vi "_Test_CRC_Calc.vi"() -> ()   [LabVIEW 2023, in "LP_CRC.lvlib"]
uses:
  LP_CRC.lvlib
panel:
  in  "Frame ID":i32=385
  out "CRC":u8=125 format="%x"
  in  "Data_In":u8[](array[numeric])=[125, 14, 64, 52, 12, 67, 49, 12, 53, 182, 13, 34, 66, 38, 86, 4, 38, 197, 29, 38, 104, 26, 34, 172, 51, 120, 150, 1, 0, 0, 0, 0, 0, 0, 0, 0, 0, 0, 0, 0, 0, 0, 0, 0, 0, 0, 0, 0, 0, 0, 0, 0, 0, 0, 0, 0, 0, 0, 0, 0, 0, 0, 0, 0] format="%x"
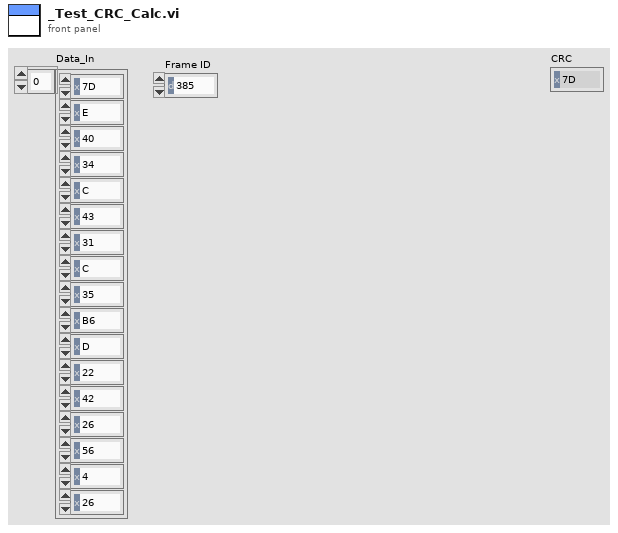
[diagram p1: front panel]
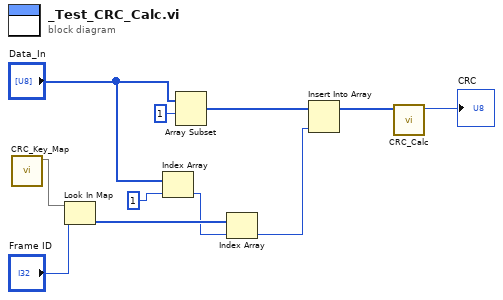
[diagram p0: block diagram]
diagram:
  n1 = call "CRC_Key_Map.vi"() -> ("Map"=w11:map{i32, u8[]})  [unwired: 11 in]
  n2 = Look In Map(map=w11, key="Frame ID") -> (value=w9:u8[])  [unwired: 1 in, 1 out]
  n3 = Index Array(array="Data_In", index=1 ("length")) -> (element=w8:u8)
  n4 = Array Subset(array="Data_In", index=1) -> (w4:u8[])  [unwired: 1 in]
  n5 = Index Array(array=w9, index=w8) -> (element=w3:u8)
  n6 = Insert Into Array(array=w4, new element=w3) -> (w2:u8[])  [unwired: 1 in]
  n7 = call "CRC_Calc.vi"("Data_in"=w2) -> ("CRC"=→"CRC":u8)  [unwired: 10 in]
